vi "Midi_SerialComm.vi"(6 "CtrlC":bool, 8 "error in (no error)":errorcluster, 9 "wait for":string, 10 "To send":string, 11 "hub":string) -> (0 "error out":errorcluster, 2 "read":string)   [LabVIEW 2022 SP3]
panel:
  out "guess":string
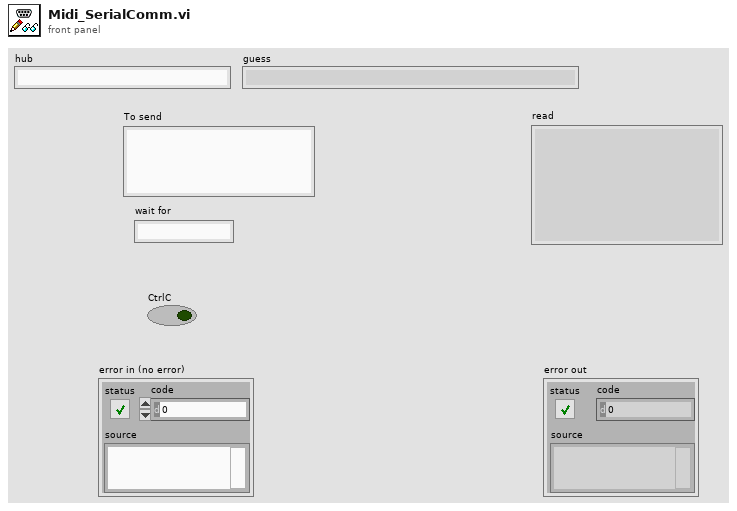
[diagram p1: front panel]
types:
  T1 = typedef "PythonCtrl.ctl" = cluster{"session":refnum<k35>, "PyPath":path, "Processor":T2, "Port":string, "version":string}
  T2 = typedef "Processors.ctl" = enum16{"SPIKE", "Pi", "Pi_ssh", "OpenMV", "Dunio"}
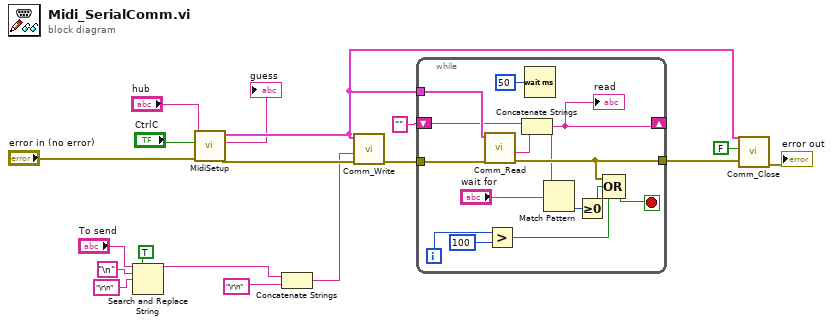
[diagram p0: block diagram]
diagram:
  n1 = Search and Replace String(replace all?=TRUE ("replace all? (F)"), input string="To send", search string="\n" ("function name"), replace string="\r\n" ("function name")) -> (result string=w5:string)  [unwired: 4 in, 3 out]
  n2 = call "MidiSetup.vi"("error in (no error)"="error in (no error)", "CtrlC"="CtrlC", "hub"="hub") -> ("error out"=w17:errorcluster, "guess"=→"guess":string, "Python"=w15:T1)  [unwired: 6 in]
  n3 = Concatenate Strings(w5, "\r\n" ("function name")) -> (w11:string)
  n4 = call "Comm_Write.vi"("error in (no error)"=w17, "Text to write"=w11, "Python"=w15) -> ("error out"=w16:errorcluster)  [unwired: 7 in, 1 out]
  n5 = while {
    tunnel: w16 -> [w32]
    tunnel: w15 -> [w31]
    tunnel: [w25] -> w14
    shift-right: [w22] -> _
    shift-left: "" -> [w29]
    i -> [w21]
    stop <- w24 stop-if-true
    n6 = call "Comm_Read.vi"("error in (no error)"=w32, "Python"=w31) -> ("error out"=w25:errorcluster, "Text read"=w30:string)  [unwired: 8 in]
    n7 = Greater?(x=w21, y=100) -> (0:w19:bool)
    n8 = Concatenate Strings(w29, w30) -> (w22:string)
    "read" <- w22
    n9 = Wait (ms)(milliseconds to wait=u32 50) -> ()  [unwired: 1 out]
    n10 = Match Pattern(string=w22, regular expression="wait for") -> (offset past match=w27:i32)  [unwired: 1 in, 3 out]
    n11 = Greater Or Equal To 0?(x=w27) -> (x >= 0?=w26:bool)
    n12 = Compound Arithmetic op=OR(w25, w26, w19) -> (w24:bool)
  }
  n13 = call "Comm_Close.vi"("error in (no error)"=w14, "Show Err?"=FALSE, "Python in"=w15) -> ("error out"=→"error out":errorcluster)  [unwired: 7 in, 1 out]
